vi "MsgBox_Win__LAVA_lib_LVTM.vi"(8 "Error in":errorcluster caption="Error in (no error)", 9 "timeout (ms)":i32=3000, 10 "strCaption":string, 11 "strText":string) -> (0 "Error out":errorcluster, 3 "Return Value":u32)   [LabVIEW 2014]
doc: "LabVIEW Task Manager v1.7.0.28\nRavi Beniwal (packaged by TimVargo) - LAVA\nCopyright (c) 2011-2014, Ravi Beniwal"
uses:
  User32.dll
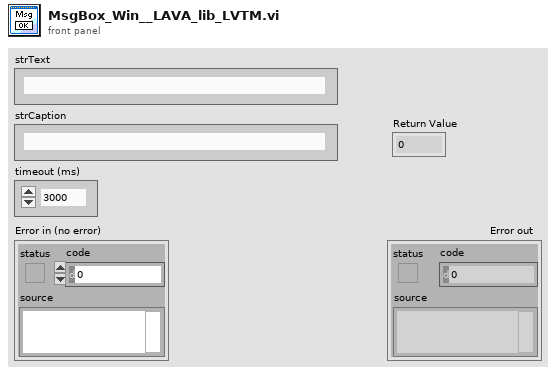
[diagram p1: front panel]
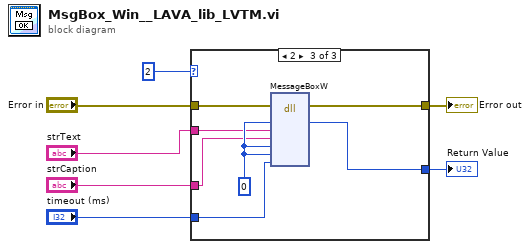
[diagram p0: block diagram]
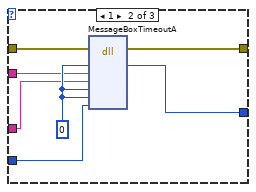
[diagram p3: hidden frame]
diagram:
  n1 = case shown="2" 2 ("NULL") {
    tunnel: "Error in" -> [w8 w15 w22]
    tunnel: [w8 w14 w21] -> w6
    tunnel: "timeout (ms)" -> [_ w12 w19]
    tunnel: [_ w11 w18] -> w4
    tunnel: "strCaption" -> [_ w10 w17]
    tunnel: "strText" -> [_ w9 w16]
    frame 0, Default {
    }
    frame 1 {
      w13 = 0 ("NULL")
      n2 = dll-call lib="user32.dll" fn="MessageBoxTimeoutA" label="MessageBoxTimeout"(error in=w15, "NULL"=w13, "strText"=w9, "strCaption"=w10, "MB_OK"=w13, "0"=w13, "sec*1000"=w12) -> (error out=w14:errorcluster, "NULL"=w11:i32)  [unwired: 8 in, 1 out]
    }
    frame 2 {
      w20 = 0 ("NULL")
      n3 = dll-call lib="user32.dll" fn="MessageBoxW" label="MessageBoxTimeout"(error in=w22, "NULL"=w20, "strText"=w16, "strCaption"=w17, "MB_OK"=w20, "0"=w20, "sec*1000"=w19) -> (error out=w21:errorcluster, "NULL"=w18:i32)  [unwired: 8 in, 1 out]
    }
  }
  "Error out" <- w6
  "Return Value" <- w4
